vi "New Stuff.vi"(6 "Conditions":T3, 7 "Overrides":T1(array[cluster]), 9 "Sample Period (s)":dbl, 10 "Limits":T2={"Velocity (fps)"=6.0, "Accel (fps^2)"=15.0, "Jerk (fps^3)"=150.0, "StoopidFast (fps)"=6.0} {"StoopidFast (fps)" min=0.0; "Jerk (fps^3)" min=0.0 step=1.0; "Accel (fps^2)" min=0.0; "Velocity (fps)" min=0.0}, 11 "Points in":cluster{"x":dbl, "y":dbl, "th":dbl}[](array[cluster])) -> (1 "result":bool)   [LabVIEW 2019]
uses:
  Limits.ctl
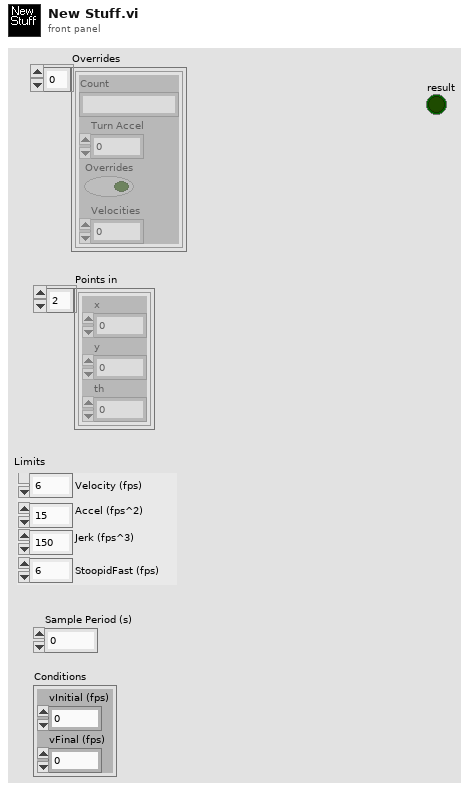
[diagram p1: front panel]
types:
  T1 = cluster{"Count":string, "Turn Accel":dbl, "Overrides":bool, "Velocities":dbl}[]
  T2 = typedef "Limits.ctl" = cluster{"Velocity (fps)":dbl, "Accel (fps^2)":dbl, "Jerk (fps^3)":dbl, "StoopidFast (fps)":dbl}
  T3 = cluster{"vInitial (fps)":dbl, "vFinal (fps)":dbl}
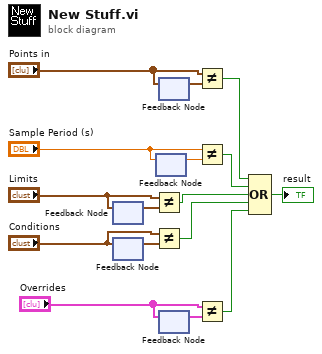
[diagram p0: block diagram]
diagram:
  n1 = feedback #1() -> (w12:T2)  [unwired: 1 in]
  n2 = feedback-in #1("Limits") -> ()
  n3 = feedback #2() -> (w14:T3)  [unwired: 1 in]
  n4 = feedback-in #2("Conditions") -> ()
  n5 = Not Equal?(x="Limits", y=w12) -> (x != y?=w4:bool)
  n6 = Not Equal?(x="Conditions", y=w14) -> (x != y?=w3:bool)
  n7 = feedback #3() -> (w8:dbl)  [unwired: 1 in]
  n8 = feedback-in #3("Sample Period (s)") -> ()
  n9 = feedback #4() -> (w10:cluster{"x":dbl, "y":dbl, "th":dbl}[])  [unwired: 1 in]
  n10 = feedback-in #4("Points in") -> ()
  n11 = feedback #5() -> (w16:T1)  [unwired: 1 in]
  n12 = feedback-in #5("Overrides") -> ()
  n13 = Not Equal?(x="Points in", y=w10) -> (x != y?=w5:bool)
  n14 = Not Equal?(x="Sample Period (s)", y=w8) -> (x != y?=w7:bool)
  n15 = Not Equal?(x="Overrides", y=w16) -> (x != y?=w2:bool)
  n16 = Compound Arithmetic op=OR(w5, w7, w4, w3, w2) -> (→"result":bool)
